vi "sub_check_connectivity.vi"(8 "error in (no error)":errorcluster, 10 "timeout (1000)":i32=1000, 11 "daq.io type in":T1={"daq.io ref"=refnum, "daq.io API Base"="http://dashboard.daq.io/api/v1", "Device Key"="", "Account ID"="", "online"=TRUE, "SSL"=FALSE}) -> (0 "error out":errorcluster, 2 "connected":bool, 3 "daq.io type out":T1={"daq.io ref"=refnum, "daq.io API Base"="http://dashboard.daq.io/api/v1", "Device Key"="", "Account ID"="", "online"=TRUE, "SSL"=FALSE})   [LabVIEW 2013, in "daqio minimal.lvlib"]
doc: "This VI \"pings\" daq.io and determines whether it can connect to it. If returning false, most likely the Internet connection is unreliable. Use this VI to regularly check for connectivity to daq.io with the least amount of traffic."
uses:
  daqio minimal.lvlib
  _typedefs/daqio-Type.ctl
  <vilib>/httpClient/ClientHandle.ctl
  _typedefs/connection_FGV_commands.ctl
  <vilib>/Easy HTTP Client/Easy HTTP.lvlib
  <vilib>/httpClient/LabVIEWHTTPClient.lvlib
panel:
  out "body":string
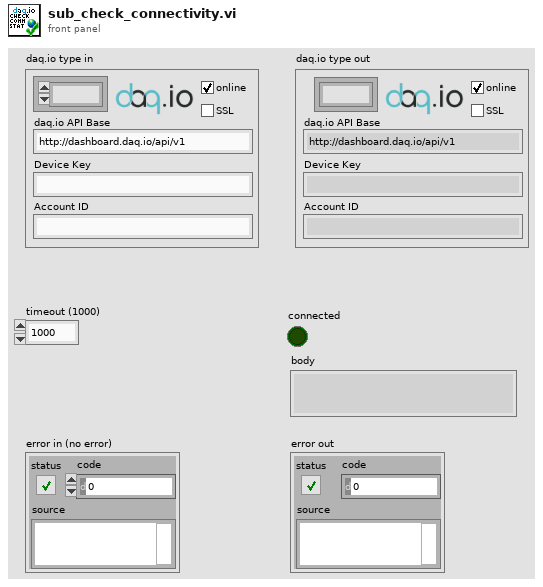
[diagram p1: front panel]
types:
  T1 = typedef "daqio minimal.lvlib/daqio-Type.ctl" = cluster{"daq.io ref":T2, "daq.io API Base":string, "Device Key":string, "Account ID":string, "online":bool, "SSL":bool}
  T2 = typedef "LabVIEWHTTPClient.lvlib/ClientHandle.ctl" = refnum<k1>
  T3 = typedef "daqio minimal.lvlib/connection_FGV_commands.ctl" = enum16{"Set Conn Stat", "Save Type", "Get Type from File", "Set Type", "Set Buffer", "Get"}
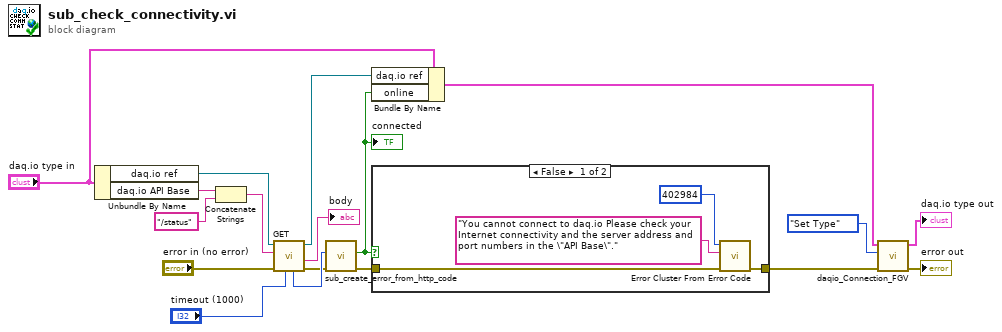
[diagram p0: block diagram]
diagram:
  n1 = Unbundle By Name("daq.io type in") -> ("daq.io ref"=w14:T2, "daq.io API Base"=w13:string)
  n2 = Concatenate Strings(w13, "/status" ("string")) -> (w17:string)
  n3 = call <vilib>:"GET.vi"("timeout (10000)"="timeout (1000)", "error in (no error)"="error in (no error)", "url"=w17, "client handle"=w14) -> ("error out"=w1:errorcluster, "body"=→"body":string, "client handle out"=w15:T2, "HTTP Response Code"=w18:i32)  [unwired: 3 in, 1 out]
  n4 = call "sub_create_error_from_http_code.vi"("error in (no error)"=w1, "HTTP Code"=w18) -> ("error out"=w4:errorcluster, "connected"=w3:bool)  [unwired: 8 in]
  "connected" <- w3
  n5 = Bundle By Name(cluster="daq.io type in", "daq.io ref"=w15, "online"=w3) -> (w6:T1)
  n6 = case shown="False" w3 {
    tunnel: w4 -> [w21 w23]
    tunnel: [w20 w23] -> w5
    frame False {
      n7 = call <vilib>:"Error Cluster From Error Code.vi"("error in (no error)"=w21, "error message (\"\")"="You cannot connect to daq.io Please check your Internet connectivity and the server address and port numbers in the \"API Base\"." ("error message (\"\")"), "error code (0)"=402984) -> ("error out"=w20:errorcluster)  [unwired: 6 in]
    }
    frame True {
    }
  }
  n8 = call "daqio_Connection_FGV.vi"("error in"=w5, "Enum"=connection_FGV_commands."Set Type", "daq.io type in"=w6) -> ("error out"=→"error out":errorcluster, "daq.io type out"=→"daq.io type out":T1)  [unwired: 5 in, 2 out]
